vi "onGetPlatanoVarietal.vi"(8 "error in (no error)":errorcluster, 11 "Banana in":refnum<class "Banana.lvclass">) -> (0 "error out":errorcluster, 2 "Varietal":string, 3 "Banana out":refnum<class "Banana.lvclass">)   [LabVIEW 2021, in "Bananas.lvlib" / "Banana.lvclass"]
uses:
  Banana.lvclass
  Banana.lvclass/Banana.ctl
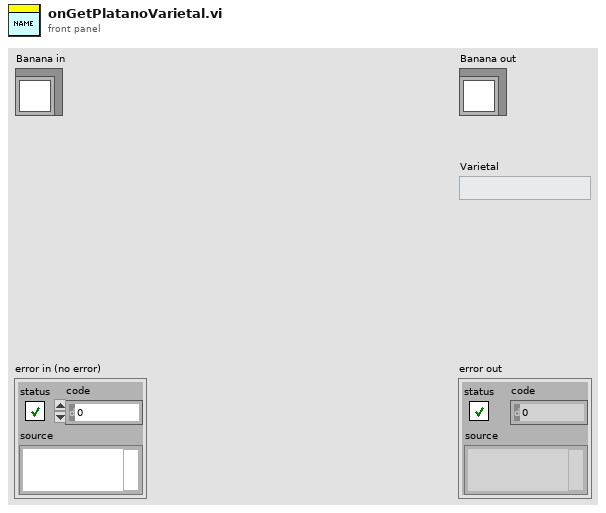
[diagram p1: front panel]
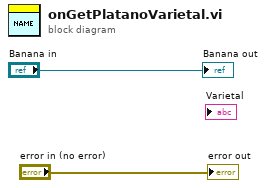
[diagram p0: block diagram]
diagram:
  "error out" <- "error in (no error)"
  "Banana out" <- "Banana in"
